vi "Dashboard Main.vi"() -> ()   [LabVIEW 2013]
uses:
  <vilib>/event_ctls.llb/eventvkey.ctl
  <vilib>/Rock Robotics/WPI/Dashboard/WPI_DashboardLogging Global.vi
  <vilib>/Utility/config.llb/Write Key (String).vi
  <vilib>/Utility/config.llb/Write Key (I32).vi
  <vilib>/Utility/config.llb/NI_LVConfig.lvlib
panel:
  out "Image Message":string="Timeout in Camera Communications"
  in  "Rec Mode":enum32{"Stop", "Record", "Playback"}(radio)
  in  "Dashboard Tab":enum32{"Main", "Test", "Checklist", "Variables"}(tab)
  in  "Camera Settings":T1={"Frame Rate"=30, "Compression"=30, "Size"=1} {"Frame Rate" scale=1.0..30.0; "Size" items=["640x480", "320x240", "160x120"]}
  out "Mode":T2(ring)=enum."Auto Disabled"
  out "Camera IP":string
  in  "DB Camera Config":bool
  out "fps":dbl format="%#.1g"
  out "Mbps":dbl format="%#.1g"
  out "Mbps 2":bool
  in  "Test Slider":dbl(slide) scale=0.0..100.0 scale format="%#_3g"
  in  "On/Off":bool caption="Solenoid"
  in  "Test Name":u16(ring) items=["Select the test to run...", "Example Test", "-------------------------------", "List of tests is built in robot code.", "Replace with your own automated tests."]
  in  "Test Tree":string(tree)
  in  "Motor":cluster{"Value":dbl, "Enable":bool} {"Value" scale=-1.0..1.0 scale format="%#_3g"}
  out "Progress":T3 {"Test Progress" scale=0.0..100.0}
  in  "Rev/Fwd":cluster{"Forward":bool, "Reverse":bool}
  in  "Test Ring":u16(ring) items=["Auto", "Fixed indoor", "Fixed outdoor 1", "Fixed outdoor 2", "Fixed fluorescent 1", "Fixed fluorescent 2", "Hold current"]
  in  "Listbox":i32(listbox)
  out "Tree":string(tree)
  out "Camera Image":T4(plugin-control)
  in  "Enable":bool
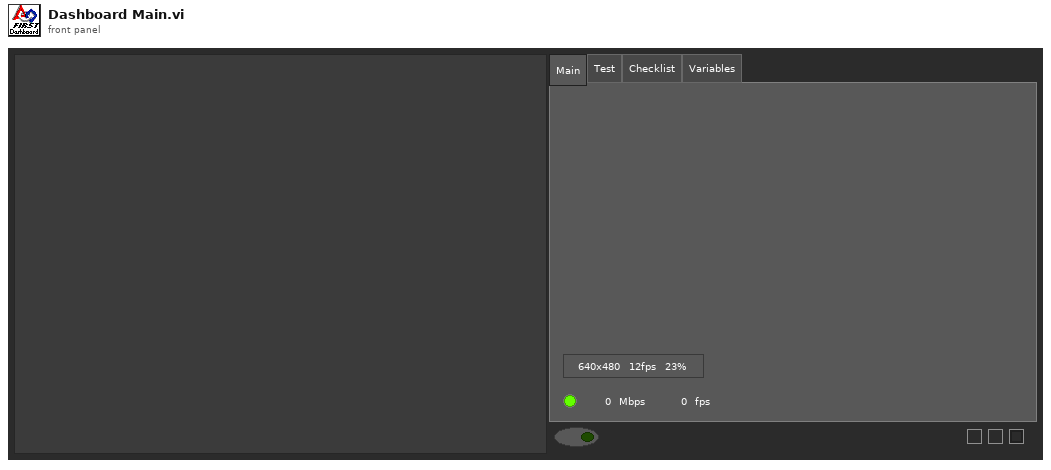
[diagram p1: front panel]
types:
  T1 = cluster{"Frame Rate":i32, "Compression":i32, "Size":u16}
  T2 = enum8{"Tele-Op Disabled", "Tele-Op Enabled", "Auto Disabled", "Auto Enabled", "Test Disabled", "Test Enabled", ""}
  T3 = cluster{"Test Progress":u8, "Test Progress Text":string}
  T4 = typedef "IMAQ Image.ctl" = refnum<image>
  T5 = enum32{"Drive", "Operation", "Auto", "Test", "Checklist", "Variables"}
  T6 = typedef "Image Type" = u32
  T7 = cluster{"Left":i32, "Top":i32, "Right":i32, "Bottom":i32}
  T8 = cluster{"Digital Inputs":bool[], "Digital Outputs":bool[]}
  T9 = cluster{"Competition mode":bool, "Robot Link":bool, "Autonomous":bool, "Enabled":bool, "E-Stop":bool, "Simulated":bool, "TestMode":bool, "Docked Window":bool}
  T10 = typedef "NI_LVConfig.lvlib/Config Data RefNum.ctl" = refnum<k1>
  T11 = typedef "eventvkey.ctl" = enum16{"ASCII", "Enter", "Return", "Shift", "Ctrl", "Alt", "Cmd", "Opt", "Caps", "NumLock", "Clear", "Break", "Up", "Down", "Left", "Right", "Insert", "Delete", "Home", "End", "PageUp", "PageDown", "Escape", "Help", "Pause", "ScrollLock", "F1", "F2", "F3", "F4", "F5", "F6", "F7", "F8", "F9", "F10", "F11", "F12", "F13", "F14", "F15", "F16", "F17", "F18", "F19", "F20", "F21", "F22", "F23", "F24", "Play", "VolumeUp", "VolumeDown", "Mute", "Two Byte Char"}
  T12 = cluster{"Image Size":bool, "Image Type":bool, "Pixel Value":bool, "ROI Information":bool, "Zoom Factor":bool}
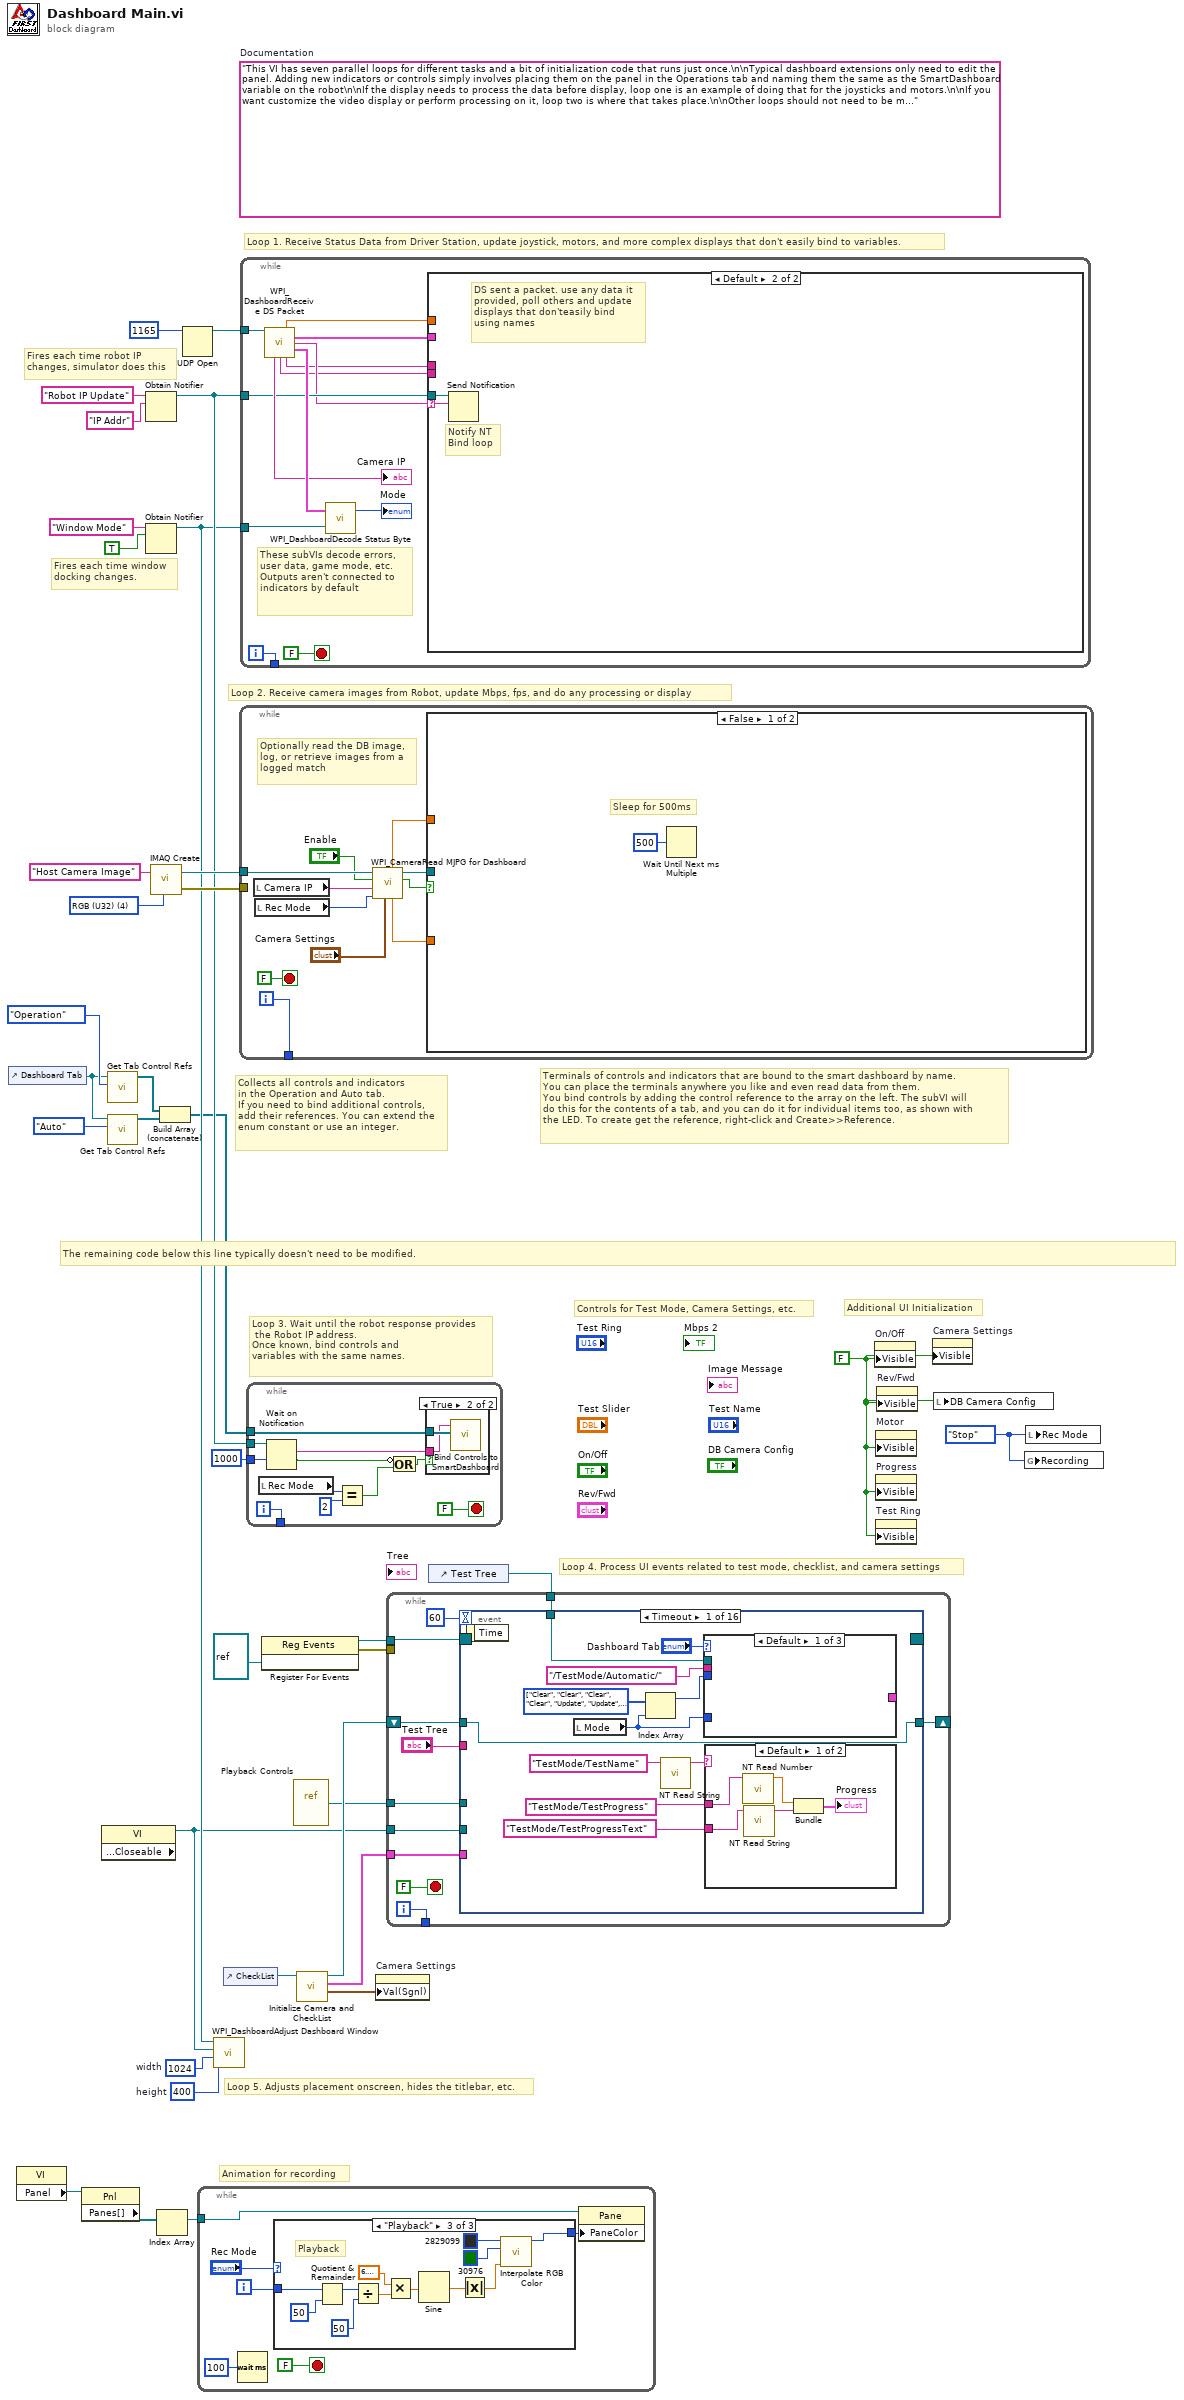
[diagram p0: block diagram]
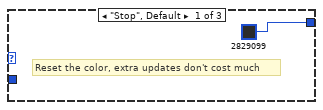
[diagram p2: hidden frame]
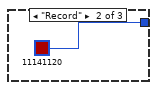
[diagram p3: hidden frame]
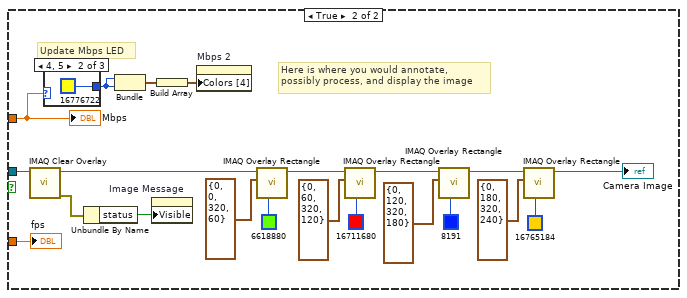
[diagram p5: hidden frame]
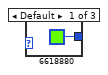
[diagram p6: hidden frame]
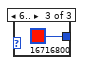
[diagram p7: hidden frame]
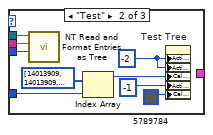
[diagram p8: hidden frame]
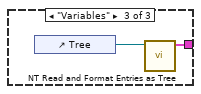
[diagram p9: hidden frame]
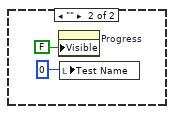
[diagram p10: hidden frame]
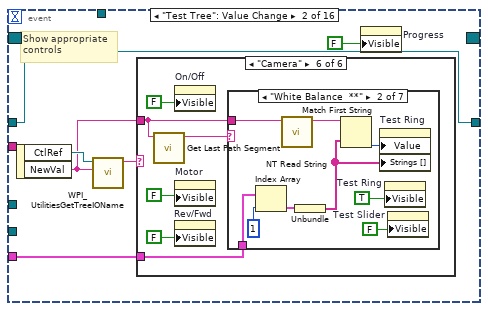
[diagram p11: hidden frame]
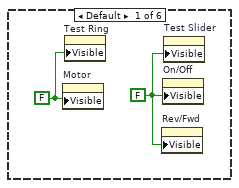
[diagram p12: hidden frame]
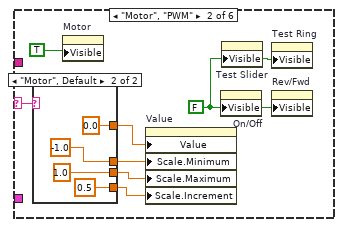
[diagram p13: hidden frame]
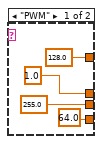
[diagram p14: hidden frame]
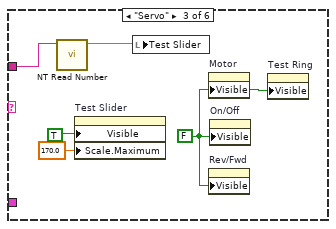
[diagram p15: hidden frame]
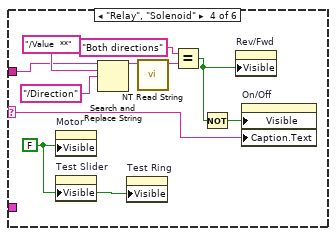
[diagram p16: hidden frame]
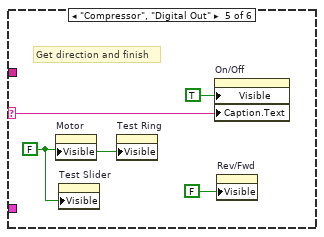
[diagram p17: hidden frame]
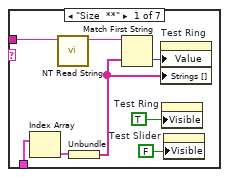
[diagram p18: hidden frame]
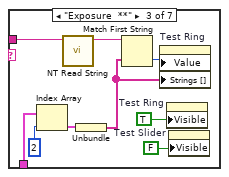
[diagram p19: hidden frame]
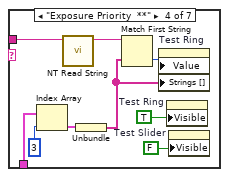
[diagram p20: hidden frame]
diagram:
  w7 = enum32{"Stop", "Record", "Playback"}."Stop" ("Rec Mode")
  w10 = 400  # height
  w11 = 1024  # width
  w24 = FALSE ("Visible")
  (unwired) "This VI has seven parallel loops for different tasks and a bit of initialization code that runs just once.\n\nTypical dashboard extensions only need to edit the panel. Adding new indicators or controls simply involves placing them on the panel in the Operations tab and naming them the same as the SmartDashboard variable on the robot\n\nIf the display needs to process the data before display, loop one is an example of doing that for the joysticks and motors.\n\nIf you want customize the video display or perform processing on it, loop two is where that takes place.\n\nOther loops should not need to be modified. They are pretty standard, and document the task they perform."  # Documentation
  w34 = T6 4 items=["Grayscale (U8)", "Grayscale (I16)", "Grayscale (SGL)", "Complex (CSG)", "RGB (U32)", "HSL (U32)", "RGB (U64)"] ("Image Type")
  # "Controls for Test Mode, Camera Settings, etc."
  # "Additional UI Initialization"
  # "Animation for recording"
  # "Fires each time robot IP\nchanges, simulator does this"
  # "Fires each time window\ndocking changes."
  # "Collects all controls and indicators\nin the Operation and Auto tab.\nIf you need to bind additional controls,\nadd their references. You can extend the\nenum constant or use an integer."
  # "The remaining code below this line typically doesn't need to be modified."
  # "Loop 4. Process UI events related to test mode, checklist, and camera settings"
  # "Terminals of controls and indicators that are bound to the smart dashboard by name.\nYou can place the terminals anywhere you like and even read data from them.\nYou bind controls by adding the control reference to the array on the left. The subVI will\ndo this for the contents of a tab, and you can do it for individual items too, as shown with\nthe LED. To create get the reference, right-click and Create>>Reference."
  # "Loop 3. Wait until the robot response provides\n the Robot IP address.\nOnce known, bind controls and\nvariables with the same names."
  # "Loop 5. Adjusts placement onscreen, hides the titlebar, etc."
  # "Loop 1. Receive Status Data from Driver Station, update joystick, motors, and more complex displays that don't easily bind to variables."
  # "Loop 2. Receive camera images from Robot, update Mbps, fps, and do any processing or display"
  n1 = control-ref of="Dashboard Tab"() -> (w5:refnum<vi>)
  n2 = property class="VI"() -> ("Panel"=w18:refnum<vi>)  [unwired: 2 in, 2 out]
  n3 = property class="Pnl"(reference=w18) -> ("Panes[]"=w19:refnum<vi>[])  [unwired: 1 in, 2 out]
  n4 = property class="VI" props=["Front Panel.Closeable"]() -> (reference out=w6:refnum<vi>)  [unwired: 2 in, 2 out]
  n5 = call <vilib>:"Get Tab Control Refs.vi"("Page Index"=T5."Operation" ("Dashboard Tab"), "TabControl in"=w5) -> ("ControlsOnPage"=w3:refnum<vi>[])  [unwired: 9 in]
  n6 = call <vilib>:"Get Tab Control Refs.vi"("Page Index"=T5."Auto" ("Dashboard Tab"), "TabControl in"=w5) -> ("ControlsOnPage"=w4:refnum<vi>[])  [unwired: 9 in]
  n7 = Obtain Notifier(name (unnamed)="Robot IP Update", notification data type="IP Addr" ("name (unnamed)")) -> (notifier out=w28:refnum<notifier>)  [unwired: 2 in, 2 out]
  n8 = Obtain Notifier(name (unnamed)="Window Mode", notification data type=TRUE) -> (notifier out=w9:refnum<notifier>)  [unwired: 2 in, 2 out]
  n9 = call "IMAQ Create"("Image Name"="Host Camera Image", "Image Type"=w34) -> ("New Image"=w32:T4, "error out"=w31:errorcluster)  [unwired: 2 in, 1 out]
  n10 = Index Array(array=w19) -> (element=w17:refnum<vi>)  [unwired: 1 in]
  n11 = Build Array (concatenate)(w3, w4) -> (w2:refnum<vi>[])
  n12 = UDP Open(11:u16 1165 ("port")) -> (port=w35:refnum<k16>)  [unwired: 2 in, 4 out]
  n13 = while {
    tunnel: w17 -> [w38]
    i -> [w41]
    stop <- FALSE stop-if-true
    n14 = Wait (ms)(milliseconds to wait=u32 100) -> ()  [unwired: 1 out]
    n15 = case shown="\"Playback\"" "Rec Mode" {
      tunnel: w41 -> [_ _ w56]
      tunnel: [u32 2829099 ("Base Color") u32 11141120 ("Target Color") w45] -> w37
      frame "Stop", Default {
        # "Reset the color, extra updates don't cost much"
      }
      frame "Record" {
      }
      frame "Playback" {
        # "Playback"
        n16 = Quotient & Remainder(x=w56, y=u32 50 ("milliseconds to wait")) -> (x-y*floor(x/y)=w52:u32)  [unwired: 1 out]
        n17 = Divide(x=w52, y=u32 50 ("milliseconds to wait")) -> (x/y=w49:dbl)
        n18 = Multiply(x=6.283185307179586, y=w49) -> (x*y=w54:dbl)
        n19 = Sine(x=w54) -> (sin(x)=w53:dbl)
        n20 = Absolute Value(x=w53) -> (abs(x)=w46:dbl)
        n21 = call "Interpolate RGB Color.vi"("Proportion"=w46, "Target Color"=u32 30976, "Base Color"=u32 2829099) -> ("Result Color"=w45:u32)  [unwired: 8 in]
      }
    }
    n22 = property class="Pane"(reference=w38, "PaneColor"=w37) -> ()  [unwired: 1 in, 2 out]
  }
  n23 = call <vilib>:"WPI_DashboardAdjust Dashboard Window.vi"("height"=w10, "width"=w11, "reference in"=w6, "Notifier in"=w9) -> ()  [unwired: 8 in]
  n24 = control-ref of="CheckList"() -> (w8:refnum<vi>)
  n25 = while {
    tunnel: w32 -> [w65]
    tunnel: w31 -> [_]
    tunnel: [w66] -> _
    i -> [w66]
    stop <- FALSE stop-if-true
    # "Optionally read the DB image,\nlog, or retrieve images from a\nlogged match"
    n26 = local read "Camera IP"() -> (w59:string)
    n27 = local read "Rec Mode"() -> (w58:enum32{"Stop", "Record", "Playback"})
    n28 = call <vilib>:"WPI_CameraRead MJPG for Dashboard.vi"("Camera Settings"="Camera Settings", "Rec Mode"=w58, "Camera IP"=w59, "Enable"="Enable", "Refnum in"=w65) -> ("Active"=w57:bool, "Refnum out"=w64:T4, "FPS"=w62:dbl, "Bandwidth (Mbps)"=w61:dbl)  [unwired: 3 in]
    n29 = case shown="False" w57 {
      tunnel: w64 -> [_ w84]
      tunnel: w61 -> [_ w83]
      tunnel: w62 -> [_ w82]
      frame False {
        # "Sleep for 500ms"
        n30 = Wait Until Next ms Multiple(millisecond multiple=u32 500) -> ()  [unwired: 1 out]
      }
      frame True {
        # "Here is where you would annotate,\npossibly process, and display the image"
        # "Update Mbps LED"
        n31 = call "IMAQ Clear Overlay"("Image"=w84) -> ("error out"=w88:errorcluster, "Image Out"=w81:T4)  [unwired: 2 in, 7 out]
        n32 = case shown="4, 5" w83 {
          tunnel: [u32 6618880 ("Color Box") u32 16776722 ("Color Box") u32 16716800 ("Color Box")] -> w85
          frame Default {
          }
          frame 4, 5 {
          }
          frame 6.. {
          }
        }
        n33 = Unbundle By Name(w88) -> ("status"=w89:bool)
        n34 = Bundle("Color Box"=w85, "Color Box"=w85) -> (w87:cluster{"Color Box":u32, "Color Box":u32})  [unwired: 1 out]
        n35 = property on="Image Message" class="Str"("Visible"=w89) -> ()  [unwired: 2 in, 2 out]
        n36 = Build Array(w87) -> (w86:cluster{"Color Box":u32, "Color Box":u32}[])
        n37 = property on="Mbps 2" class="Bool (strict)"("Colors [4]"=w86) -> ()  [unwired: 2 in, 2 out]
        n38 = call "IMAQ Overlay Rectangle"("Color"=u32 6618880, "Rectangle"=T7 {"Left"=0, "Top"=0, "Right"=320, "Bottom"=60}, "Image"=w81) -> ("Image Out"=w80:T4)  [unwired: 7 in, 1 out]
        n39 = call "IMAQ Overlay Rectangle"("Color"=u32 16711680, "Rectangle"=T7 {"Left"=0, "Top"=60, "Right"=320, "Bottom"=120}, "Image"=w80) -> ("Image Out"=w79:T4)  [unwired: 7 in, 1 out]
        n40 = call "IMAQ Overlay Rectangle"("Color"=u32 8191, "Rectangle"=T7 {"Left"=0, "Top"=120, "Right"=320, "Bottom"=180}, "Image"=w79) -> ("Image Out"=w78:T4)  [unwired: 7 in, 1 out]
        n41 = call "IMAQ Overlay Rectangle"("Color"=u32 16765184, "Rectangle"=T7 {"Left"=0, "Top"=180, "Right"=320, "Bottom"=240}, "Image"=w78) -> ("Image Out"=→"Camera Image":T4)  [unwired: 7 in, 1 out]
        "Mbps" <- w83
        "fps" <- w82
      }
    }
  }
  n42 = while {
    tunnel: w35 -> [w103]
    tunnel: w28 -> [w98]
    tunnel: w9 -> [w102]
    tunnel: [w99] -> _
    i -> [w99]
    stop <- FALSE stop-if-true
    # "These subVIs decode errors, user data, game mode, etc.\nOutputs aren't connected to indicators by default"
    n43 = call <vilib>:"WPI_DashboardReceive DS Packet.vi"("Recv Socket"=w103) -> ("Battery"=w93:sgl, "Driver Station"=w94:T8, "Robot IP Address"=w97:string, "Status"=w104:T9, "Camera IP Address"=→"Camera IP":string, "Low Priority User Data"=w96:string, "High Priority User Data"=w95:string)  [unwired: 1 in, 7 out]
    n44 = call <vilib>:"WPI_DashboardDecode Status Byte.vi"("Window Mode Notifier"=w102, "Status"=w104) -> ("Mode"=→"Mode":T2)  [unwired: 1 out]
    n45 = case shown="Default" w97 {
      selector: w97 -> [_ w106]
      tunnel: w98 -> [_ w107]
      tunnel: w96 -> [_ _]
      tunnel: w95 -> [_ _]
      tunnel: w94 -> [_ _]
      tunnel: w93 -> [_ _]
      frame "0.0.0.0" {
        # "DS not sending packets, or no robot exists yet.\nDon't poll the variables"
      }
      frame Default {
        # "Notify NT\nBind loop"
        # "DS sent a packet. use any data it\nprovided, poll others and update\ndisplays that don'teasily bind\nusing names"
        n46 = Send Notification(notification=w106, notifier=w107) -> ()  [unwired: 1 in, 2 out]
      }
    }
  }
  n47 = while {
    tunnel: w2 -> [w118]
    tunnel: w28 -> [w116]
    tunnel: [w114] -> _
    tunnel: u32 1000 ("milliseconds to wait") -> [w113]
    i -> [w114]
    stop <- FALSE stop-if-true
    n48 = local read "Rec Mode"() -> (w109:enum32{"Stop", "Record", "Playback"})
    n49 = Wait on Notification(notifier=w116, timeout in ms (-1)=w113) -> (notification=w115:string, timed out?=w111:bool)  [unwired: 2 in, 2 out]
    n50 = Equal?(x=w109, y=u16 2 ("Rec Mode")) -> (x = y?=w110:bool)
    n51 = Compound Arithmetic op=OR(invert w111, w110) -> (w112:bool)
    n52 = case shown="True" w112 {
      tunnel: w118 -> [_ w120]
      tunnel: w115 -> [_ w119]
      frame False {
      }
      frame True {
        n53 = call <vilib>:"Bind Controls to SmartDashboard.vi"("Bound Control Refs"=w120, "Server IP Address"=w119) -> ()  [unwired: 10 in]
      }
    }
  }
  n54 = register-events(refnum<vi> refnum) -> (reference out=w15:refnum<event-registration>, error out=w14:errorcluster)  [unwired: 2 in]
  n55 = vi-ref "Playback Controls.vi"() -> (w16:refnum<vi>)
  n56 = call "Initialize Camera and CheckList.vi"("ListBox in"=w8) -> ("Cluster"=w22:cluster{"value":i32, "value":i32, "index":i32}, "Array"=w23:cluster{string[]}[], "File Refnum"=w21:T10)  [unwired: 8 in]
  n57 = property on="Camera Settings" class="Clust (strict)"("Val(Sgnl)"=w22) -> ()  [unwired: 2 in, 2 out]
  n58 = control-ref of="Test Tree"() -> (w20:refnum<vi>)
  n59 = while {
    tunnel: w23 -> [w128]
    shift-right: [w127] -> _
    shift-left: w21 -> [w126]
    tunnel: [w125] -> _
    tunnel: w20 -> [w124]
    tunnel: w16 -> [w123]
    tunnel: w15 -> [w122]
    tunnel: w14 -> [_]
    tunnel: w6 -> [w121]
    i -> [w125]
    stop <- FALSE stop-if-true
    n60 = event shown="[0] Timeout" {
      selector: w122 -> [_ _ _ _ _ _ _ _ _ _ _ _ _ _ _ _]
      dyn-events: [_ _ _ _ _ _ _ _ _ _ _ _ _ w366 _ _] -> _
      timeout: u32 60 ("milliseconds to wait") -> [_ _ _ _ _ _ _ _ _ _ _ _ _ _ _ _]
      tunnel: w124 -> [w138 _ _ _ _ _ _ _ _ _ _ _ _ _ _ _]
      tunnel: "Test Tree" -> [_ _ _ _ _ _ _ _ w335 w343 w345 w349 w357 _ _ _]
      tunnel: w128 -> [_ w162 _ _ _ _ w299 w329 _ _ _ _ _ _ _ _]
      tunnel: [w132 w161 w260 w265 w273 w285 w298 w322 w334 w341 w344 w348 w356 w368 w382 w383] -> w127
      tunnel: w126 -> [w132 w161 w260 w265 w273 w285 w297 w322 w334 w341 w344 w348 w356 w368 w382 w383]
      tunnel: w123 -> [_ _ _ _ _ _ _ _ _ _ _ _ _ w369 _ w386]
      tunnel: w121 -> [_ _ _ _ _ _ _ _ _ _ _ _ _ w364 _ _]
      event Timeout {
        w137 = enum16{"Update", "Clear"}[] [enum."Clear", enum."Clear", enum."Clear", enum."Clear", enum."Update", enum."Update", enum."Clear"] items=["Update", "Clear"]
        n61 = event-data() -> ()  [unwired: 1 in, 1 out]
        n62 = local read "Mode"() -> (w135:T2)
        n63 = Index Array(array=w137, index=w135) -> (element=w136:enum16{"Update", "Clear"})
        n64 = call <vilib>:"NT Read String.vi"("Name"="TestMode/TestName") -> ("String"=w141:string)  [unwired: 9 in, 1 out]
        n65 = case shown="Default" "Dashboard Tab" {
          tunnel: w138 -> [_ w151 _]
          tunnel: "/TestMode/Automatic/" ("Name Pattern") -> [_ w150 _]
          tunnel: w136 -> [_ w149 _]
          tunnel: w135 -> [_ w147 _]
          tunnel: [_ _ w153] -> _
          frame Default {
          }
          frame "Test" {
            w146 = -2 ("Active Item:Row Number")
            n66 = call <vilib>:"NT Read and Format Entries as Tree.vi"("Operation"=w149, "Name Pattern"=w150, "Tree Refnum"=w151) -> ()  [unwired: 7 in, 2 out]
            n67 = Index Array(array=u32[] [14013909, 14013909, 14013909, 14013909, 14013909, 16777215, 14013909], index=w147) -> (element=w145:u32)
            n68 = property on="Test Tree" class="Tree (strict)"("Active Item Row Number"=w146, "ActiveColNum"=w146, "CellBG"=w145, "Active Item Row Number"=-1 ("Active Item:Row Number"), "CellBG"=u32 5789784 ("Color Box")) -> ()  [unwired: 2 in, 2 out]
          }
          frame "Variables" {
            n69 = control-ref of="Tree"() -> (w152:refnum<vi>)
            n70 = call <vilib>:"NT Read and Format Entries as Tree.vi"("Tree Refnum"=w152) -> ("Formatted Strings"=w153:cluster{"Name":string, "Value":string}[])  [unwired: 9 in, 1 out]
          }
        }
        n71 = case shown="Default" w141 {
          tunnel: "TestMode/TestProgress" ("Name") -> [w155 _]
          tunnel: "TestMode/TestProgressText" ("Name") -> [w154 _]
          frame Default {
            n72 = call <vilib>:"NT Read Number.vi"("Name"=w155) -> ("Numeric"=w156:dbl)  [unwired: 9 in, 1 out]
            n73 = call <vilib>:"NT Read String.vi"("Name"=w154) -> ("String"=w157:string)  [unwired: 9 in, 1 out]
            n74 = Bundle("Numeric"=w156, "String"=w157) -> (→"Progress":cluster{"Numeric":dbl, "String":string})  [unwired: 1 in]
          }
          frame "" {
            n75 = property on="Progress" class="Clust (strict)"("Visible"=FALSE) -> ()  [unwired: 2 in, 2 out]
            n76 = local write "Test Name"(u16 0) -> ()
          }
        }
      }
      event "Test Tree": Value Change {
        # "Show appropriate\ncontrols"
        n77 = event-data() -> ("CtlRef"=w165:refnum<vi>, "NewVal"=w163:string)  [unwired: 1 in]
        n78 = call <vilib>:"WPI_UtilitiesGetTreeIOName.vi"("NewVal"=w163, "TreeControl in"=w165) -> ("I/O Name"=w166:string)  [unwired: 9 in]
        n79 = case shown="\"Camera\"" w166 {
          selector: w166 -> [_ w173 _ w191 w200 _]
          tunnel: w163 -> [_ _ w188 w190 _ w207]
          tunnel: w162 -> [_ _ _ _ _ w206]
          frame Default {
            w168 = FALSE ("Visible")
            w167 = FALSE ("Visible")
            n80 = property on="Motor" class="Clust (strict)"("Visible"=w167) -> ()  [unwired: 2 in, 2 out]
            n81 = property on="Test Ring" class="Ring (strict)"("Visible"=w167) -> ()  [unwired: 2 in, 2 out]
            n82 = property on="Rev/Fwd" class="Clust (strict)"("Visible"=w168) -> ()  [unwired: 2 in, 2 out]
            n83 = property on="On/Off" class="Bool (strict)"("Visible"=w168) -> ()  [unwired: 2 in, 2 out]
            n84 = property on="Test Slider" class="Slide (strict)"("Visible"=w168) -> ()  [unwired: 2 in, 2 out]
          }
          frame "Motor", "PWM" {
            w174 = FALSE ("Visible")
            n85 = case shown="\"Motor\", Default" w173 {
              tunnel: [1.0 ("Value") -1.0 ("Value")] -> w172
              tunnel: [255.0 ("Value") 1.0 ("Value")] -> w171
              tunnel: [128.0 ("Value") 0.0 ("Value")] -> w170
              tunnel: [64.0 ("Value") 0.5 ("Value")] -> w169
              frame "PWM" {
              }
              frame "Motor", Default {
              }
            }
            n86 = property on="Motor" class="Clust (strict)"("Visible"=TRUE) -> ()  [unwired: 2 in, 2 out]
            n87 = property on="Value" class="Slide (strict)"("Value"=w170, "Scale.Minimum"=w172, "Scale.Maximum"=w171, "Scale.Increment"=w169) -> ()  [unwired: 2 in, 2 out]
            n88 = property on="On/Off" class="Bool (strict)"("Visible"=w174) -> ()  [unwired: 2 in, 2 out]
            n89 = property on="Test Slider" class="Slide (strict)"("Visible"=w174) -> ()  [unwired: 2 in, 2 out]
            n90 = property on="Test Ring" class="Ring (strict)"("Visible"=w174) -> ()  [unwired: 2 in, 2 out]
            n91 = property on="Rev/Fwd" class="Clust (strict)"("Visible"=w174) -> ()  [unwired: 2 in, 2 out]
          }
          frame "Servo" {
            w186 = FALSE ("Visible")
            n92 = call <vilib>:"NT Read Number.vi"("Name"=w188) -> ("Numeric"=w187:dbl)  [unwired: 9 in, 1 out]
            n93 = property on="Test Slider" class="Slide (strict)"("Visible"=TRUE, "Scale.Maximum"=170.0 ("Scale.Range:Maximum")) -> ()  [unwired: 2 in, 2 out]
            n94 = local write "Test Slider"(w187) -> ()
            n95 = property on="Motor" class="Clust (strict)"("Visible"=w186) -> ()  [unwired: 2 in, 2 out]
            n96 = property on="Rev/Fwd" class="Clust (strict)"("Visible"=w186) -> ()  [unwired: 2 in, 2 out]
            n97 = property on="On/Off" class="Bool (strict)"("Visible"=w186) -> ()  [unwired: 2 in, 2 out]
            n98 = property on="Test Ring" class="Ring (strict)"("Visible"=w186) -> ()  [unwired: 2 in, 2 out]
          }
          frame "Relay", "Solenoid" {
            w189 = FALSE ("Visible")
            n99 = property on="Motor" class="Clust (strict)"("Visible"=w189) -> ()  [unwired: 2 in, 2 out]
            n100 = property on="Test Slider" class="Slide (strict)"("Visible"=w189) -> ()  [unwired: 2 in, 2 out]
            n101 = Search and Replace String(input string=w190, search string="/Value  **", replace string="/Direction") -> (result string=w196:string)  [unwired: 5 in, 3 out]
            n102 = property on="Test Ring" class="Ring (strict)"("Visible"=w189) -> ()  [unwired: 2 in, 2 out]
            n103 = call <vilib>:"NT Read String.vi"("Name"=w196) -> ("String"=w194:string)  [unwired: 9 in, 1 out]
            n104 = Equal?(x="Both directions", y=w194) -> (x = y?=w192:bool)
            n105 = Not(x=w192) -> (.not. x?=w193:bool)
            n106 = property on="Rev/Fwd" class="Clust (strict)"("Visible"=w192) -> ()  [unwired: 2 in, 2 out]
            n107 = property on="On/Off" class="Bool (strict)"("Visible"=w193, "Caption.Text"=w191) -> ()  [unwired: 2 in, 2 out]
          }
          frame "Compressor", "Digital Out" {
            w199 = FALSE ("Visible")
            # "Get direction and finish"
            n108 = property on="Motor" class="Clust (strict)"("Visible"=w199) -> ()  [unwired: 2 in, 2 out]
            n109 = property on="Test Slider" class="Slide (strict)"("Visible"=w199) -> ()  [unwired: 2 in, 2 out]
            n110 = property on="Test Ring" class="Ring (strict)"("Visible"=w199) -> ()  [unwired: 2 in, 2 out]
            n111 = property on="On/Off" class="Bool (strict)"("Visible"=TRUE, "Caption.Text"=w200) -> ()  [unwired: 2 in, 2 out]
            n112 = property on="Rev/Fwd" class="Clust (strict)"("Visible"=FALSE) -> ()  [unwired: 2 in, 2 out]
          }
          frame "Camera" {
            n113 = call <vilib>:"Get Last Path Segment.vi"("String in"=w207) -> ("String out"=w208:string)  [unwired: 10 in]
            n114 = property on="On/Off" class="Bool (strict)"("Visible"=FALSE) -> ()  [unwired: 2 in, 2 out]
            n115 = property on="Motor" class="Clust (strict)"("Visible"=FALSE) -> ()  [unwired: 2 in, 2 out]
            n116 = property on="Rev/Fwd" class="Clust (strict)"("Visible"=FALSE) -> ()  [unwired: 2 in, 2 out]
            n117 = case shown="\"White Balance  **\"" w208 {
              tunnel: w207 -> [w214 w223 w232 w241 w250 _ w256]
              tunnel: w206 -> [w212 w220 w229 w238 w247 _ _]
              frame "Size  **" {
                n118 = Index Array(array=w212) -> (element=w211:cluster{string[]})  [unwired: 1 in]
                n119 = call <vilib>:"NT Read String.vi"("Name"=w214) -> ("String"=w213:string)  [unwired: 9 in, 1 out]
                n120 = Unbundle(w211) -> (w209:string[])
                n121 = Match First String(2:w209, 3:w213) -> (0:w210:i32)  [unwired: 1 out]
                n122 = property on="Test Ring" class="Ring (strict)"("Value"=w210, "Strings []"=w209) -> ()  [unwired: 2 in, 2 out]
                n123 = property on="Test Ring" class="Ring (strict)"("Visible"=TRUE) -> ()  [unwired: 2 in, 2 out]
                n124 = property on="Test Slider" class="Slide (strict)"("Visible"=FALSE) -> ()  [unwired: 2 in, 2 out]
              }
              frame "White Balance  **" {
                n125 = Index Array(array=w220, index=1) -> (element=w221:cluster{string[]})
                n126 = call <vilib>:"NT Read String.vi"("Name"=w223) -> ("String"=w222:string)  [unwired: 9 in, 1 out]
                n127 = Unbundle(w221) -> (w218:string[])
                n128 = Match First String(2:w218, 3:w222) -> (0:w217:i32)  [unwired: 1 out]
                n129 = property on="Test Ring" class="Ring (strict)"("Value"=w217, "Strings []"=w218) -> ()  [unwired: 2 in, 2 out]
                n130 = property on="Test Ring" class="Ring (strict)"("Visible"=TRUE) -> ()  [unwired: 2 in, 2 out]
                n131 = property on="Test Slider" class="Slide (strict)"("Visible"=FALSE) -> ()  [unwired: 2 in, 2 out]
              }
              frame "Exposure  **" {
                n132 = Index Array(array=w229, index=2) -> (element=w230:cluster{string[]})
                n133 = call <vilib>:"NT Read String.vi"("Name"=w232) -> ("String"=w231:string)  [unwired: 9 in, 1 out]
                n134 = Unbundle(w230) -> (w226:string[])
                n135 = Match First String(2:w226, 3:w231) -> (0:w227:i32)  [unwired: 1 out]
                n136 = property on="Test Ring" class="Ring (strict)"("Value"=w227, "Strings []"=w226) -> ()  [unwired: 2 in, 2 out]
                n137 = property on="Test Ring" class="Ring (strict)"("Visible"=TRUE) -> ()  [unwired: 2 in, 2 out]
                n138 = property on="Test Slider" class="Slide (strict)"("Visible"=FALSE) -> ()  [unwired: 2 in, 2 out]
              }
              frame "Exposure Priority  **" {
                n139 = Index Array(array=w238, index=3) -> (element=w239:cluster{string[]})
                n140 = call <vilib>:"NT Read String.vi"("Name"=w241) -> ("String"=w240:string)  [unwired: 9 in, 1 out]
                n141 = Unbundle(w239) -> (w235:string[])
                n142 = Match First String(2:w235, 3:w240) -> (0:w236:i32)  [unwired: 1 out]
                n143 = property on="Test Ring" class="Ring (strict)"("Value"=w236, "Strings []"=w235) -> ()  [unwired: 2 in, 2 out]
                n144 = property on="Test Ring" class="Ring (strict)"("Visible"=TRUE) -> ()  [unwired: 2 in, 2 out]
                n145 = property on="Test Slider" class="Slide (strict)"("Visible"=FALSE) -> ()  [unwired: 2 in, 2 out]
              }
              frame "Color Enable  **" {
                n146 = Index Array(array=w247, index=4) -> (element=w248:cluster{string[]})
                n147 = call <vilib>:"NT Read String.vi"("Name"=w250) -> ("String"=w249:string)  [unwired: 9 in, 1 out]
                n148 = Unbundle(w248) -> (w244:string[])
                n149 = Match First String(2:w244, 3:w249) -> (0:w245:i32)  [unwired: 1 out]
                n150 = property on="Test Ring" class="Ring (strict)"("Value"=w245, "Strings []"=w244) -> ()  [unwired: 2 in, 2 out]
                n151 = property on="Test Ring" class="Ring (strict)"("Visible"=TRUE) -> ()  [unwired: 2 in, 2 out]
                n152 = property on="Test Slider" class="Slide (strict)"("Visible"=FALSE) -> ()  [unwired: 2 in, 2 out]
              }
              frame Default {
                n153 = property on="Test Ring" class="Ring (strict)"("Visible"=FALSE) -> ()  [unwired: 2 in, 2 out]
                n154 = property on="Test Slider" class="Slide (strict)"("Visible"=FALSE) -> ()  [unwired: 2 in, 2 out]
              }
              frame "Brightness  **", "Color Level  **", "Compression  **", "FPS  **", "Sharpness  **" {
                n155 = call <vilib>:"NT Read Number.vi"("Name"=w256) -> ("Numeric"=w255:dbl)  [unwired: 9 in, 1 out]
                n156 = local write "Test Slider"(w255) -> ()
                n157 = property on="Test Slider" class="Slide (strict)"("Visible"=TRUE, "Scale.Maximum"=100.0 ("Scale.Range:Maximum")) -> ()  [unwired: 2 in, 2 out]
                n158 = property on="Test Ring" class="Ring (strict)"("Visible"=FALSE) -> ()  [unwired: 2 in, 2 out]
              }
            }
          }
        }
        n159 = property on="Progress" class="Clust (strict)"("Visible"=FALSE) -> ()  [unwired: 2 in, 2 out]
      }
      event "Test Name": Mouse Enter {
        # "Populate the ring with the list of tests"
        n160 = event-data() -> ()  [unwired: 1 in, 1 out]
        n161 = call <vilib>:"NT Read String Array.vi"("Name"="TestMode/TestList") -> ("String Array"=w264:string[])  [unwired: 9 in, 1 out]
        n162 = Build Array (concatenate)("Select the test to run...", w264) -> (w263:string[])
        n163 = property on="Test Name" class="Ring (strict)"("Strings []"=w263) -> ()  [unwired: 2 in, 2 out]
      }
      event "Test Name": Value Change {
        w266 = FALSE ("Visible")
        # "Tell the robot the test name to run"
        n164 = event-data() -> ("NewVal"=w270:u16)  [unwired: 1 in]
        n165 = property on="Test Name" class="Ring (strict)"() -> ("Strings []"=w271:string[])  [unwired: 2 in, 2 out]
        n166 = local write "Progress"(T3 {"Test Progress"=0, "Test Progress Text"=""} ("Progress")) -> ()
        n167 = Index Array(array=w271, index=w270) -> (element=w269:string)
        n168 = call <vilib>:"NT Write String.vi"("String"=w269, "Name"="TestMode/TestName") -> ()  [unwired: 9 in, 1 out]
        n169 = property on="Progress" class="Clust (strict)"("Visible"=TRUE) -> ()  [unwired: 2 in, 2 out]
        n170 = property on="Motor" class="Clust (strict)"("Visible"=w266) -> ()  [unwired: 2 in, 2 out]
        n171 = property on="Test Slider" class="Slide (strict)"("Visible"=w266) -> ()  [unwired: 2 in, 2 out]
        n172 = property on="On/Off" class="Bool (strict)"("Visible"=w266) -> ()  [unwired: 2 in, 2 out]
        n173 = property on="Rev/Fwd" class="Clust (strict)"("Visible"=w266) -> ()  [unwired: 2 in, 2 out]
        n174 = property on="Test Ring" class="Ring (strict)"("Visible"=w266) -> ()  [unwired: 2 in, 2 out]
      }
      event "Listbox": Double Click {
        n175 = event-data() -> ("PlatMods.Shift"=w274:bool, "Row"=w276:i32)  [unwired: 1 in]
        n176 = case shown="True" w274 {
          tunnel: w276 -> [w280 _]
          tunnel: 1 -> [w279 _]
          frame False {
            n177 = property on="Listbox" class="LstBox (strict)"() -> ("Item Symbols"=w278:i32[])  [unwired: 2 in, 2 out]
            n178 = Replace Array Subset(array=w278, new element=w279, index=w280) -> (w277:i32[])
            n179 = property on="Listbox" class="LstBox (strict)"("Item Symbols"=w277) -> ()  [unwired: 2 in, 2 out]
          }
          frame True {
            w281 = 0 ("Top Row")
            n180 = property on="Listbox" class="LstBox (strict)"() -> ("Number of Rows"=w283:u32)  [unwired: 2 in, 2 out]
            n181 = Initialize Array(0, w283) -> (w282:i32[])
            n182 = property on="Listbox" class="LstBox (strict)"("Top Row"=w281, "Value"=w281, "Item Symbols"=w282) -> ()  [unwired: 2 in, 2 out]
          }
        }
      }
      event "Listbox": Key Down {
        n183 = event-data() -> ("VKey"=w287:T11)  [unwired: 1 in]
        n184 = case shown="\"Left\", \"Right\"" w287 {
          selector: w287 -> [w292 _]
          tunnel: eventvkey."Left" ("VKey") -> [w290 _]
          frame "Left", "Right" {
            n185 = Equal?(x=w290, y=w292) -> (x = y?=w291:bool)
            n186 = Select(t=0, s=w291, f=1) -> (s? t:f=w293:i32)
            n187 = property on="Listbox" class="LstBox (strict)"() -> ("Item Symbols"=w296:i32[])  [unwired: 2 in, 2 out]
            n188 = Replace Array Subset(array=w296, new element=w293, index="Listbox") -> (w295:i32[])
            n189 = property on="Listbox" class="LstBox (strict)"("Item Symbols"=w295) -> ()  [unwired: 2 in, 2 out]
          }
          frame Default {
          }
        }
      }
      event "DB Camera Config": Value Change {
        n190 = event-data() -> ("NewVal"=w300:bool)  [unwired: 1 in]
        n191 = case shown="False" w300 {
          tunnel: w299 -> [w309 _]
          tunnel: [w302 w320] -> w298
          tunnel: w297 -> [w301 w320]
          frame False {
            w316 = "Camera"
            w319 = FALSE ("Visible")
            n192 = local read "Camera Settings"() -> (w308:T1)
            n193 = Index Array(array=w309) -> (element=w312:cluster{string[]})  [unwired: 1 in]
            n194 = Unbundle(w308) -> ("Frame Rate"=w307:i32, "Compression"=w306:i32, "Size"=w310:u16)
            n195 = Unbundle(w312) -> (w311:string[])
            n196 = Index Array(array=w311, index=w310) -> (element=w305:string)
            n197 = call-poly <vilib>:"Write Key.vi"("section"=w316, "value"=w305, "key"="Size", "refnum"=w301) -> ("refnum out"=w318:T10)  [unwired: 2 in, 5 out]
            n198 = call-poly <vilib>:"Write Key.vi"("section"=w316, "value"=w307, "key"="FrameRate", "refnum"=w318) -> ("refnum out"=w317:T10)  [unwired: 1 in, 6 out]
            n199 = property on="Camera Settings" class="Clust (strict)"("Visible"=w319) -> ()  [unwired: 2 in, 2 out]
            n200 = local write "DB Camera Config"(w319) -> ()
            n201 = call-poly <vilib>:"Write Key.vi"("section"=w316, "value"=w306, "key"="Compression", "refnum"=w317) -> ("refnum out"=w303:T10)  [unwired: 1 in, 6 out]
            n202 = call <vilib>:"Close Config Data.vi"("refnum"=w303) -> ("file path"=w304:path)  [unwired: 2 in, 8 out]
            n203 = call <vilib>:"Open Config Data.vi"("configuration file path"=w304) -> ("refnum"=w302:T10)  [unwired: 8 in, 2 out]
          }
          frame True {
            n204 = property on="Camera Settings" class="Clust (strict)"("Visible"=TRUE) -> ()  [unwired: 2 in, 2 out]
          }
        }
      }
      event "Camera Settings": Value Change {
        n205 = event-data() -> ("NewVal"=w333:T1)  [unwired: 1 in]
        n206 = Index Array(array=w329) -> (element=w328:cluster{string[]})  [unwired: 1 in]
        n207 = Unbundle(w333) -> ("Frame Rate"=w324:i32, "Compression"=w323:i32, "Size"=w326:u16)
        n208 = Unbundle(w328) -> (w327:string[])
        n209 = Index Array(array=w327, index=w326) -> (element=w325:string)
        n210 = Format Into String(format string="%s   %dfps   %d%%", w325, w324, w323) -> (resulting string=w330:string)  [unwired: 2 in, 1 out]
        n211 = Build Array(w330) -> (w331:string[])
        n212 = property on="DB Camera Config" class="Bool (strict)"("Strings [4]"=w331) -> ()  [unwired: 2 in, 2 out]
      }
      event "Motor.Enable": Value Change {
        n213 = event-data() -> ("NewVal"=w339:bool)  [unwired: 1 in]
        n214 = Unbundle("Motor") -> ("Value"=w338:dbl)  [unwired: 1 out]
        n215 = Select(t=w338, s=w339, f=0.0) -> (s? t:f=w336:dbl)
        n216 = call <vilib>:"NT Write Number.vi"("Numeric"=w336, "Name"=w335) -> ()  [unwired: 9 in, 1 out]
      }
      event "Test Slider": Value Change {
        n217 = event-data() -> ("NewVal"=w342:dbl)  [unwired: 1 in]
        n218 = call <vilib>:"NT Write Number.vi"("Numeric"=w342, "Name"=w343) -> ()  [unwired: 9 in, 1 out]
      }
      event "On/Off": Value Change {
        n219 = event-data() -> ("NewVal"=w347:bool)  [unwired: 1 in]
        n220 = Boolean To (0,1)(Boolean=w347) -> (0, 1=w346:i16)
        n221 = call <vilib>:"NT Write Number.vi"("Numeric"=w346, "Name"=w345) -> ()  [unwired: 9 in, 1 out]
      }
      event "Rev/Fwd": Value Change {
        n222 = event-data() -> ("NewVal.Forward"=w355:bool, "NewVal.Reverse"=w354:bool)  [unwired: 1 in]
        n223 = Boolean To (0,1)(Boolean=w355) -> (0, 1=w351:i16)
        n224 = Boolean To (0,1)(Boolean=w354) -> (0, 1=w353:i16)
        n225 = Negate(x=w353) -> (-x=w352:i16)
        n226 = Add(x=w351, y=w352) -> (x+y=w350:i16)
        n227 = call <vilib>:"NT Write Number.vi"("Numeric"=w350, "Name"=w349) -> ()  [unwired: 9 in, 1 out]
      }
      event "Test Ring": Value Change {
        n228 = event-data() -> ("NewVal"=w359:u16)  [unwired: 1 in]
        n229 = property on="Test Ring" class="Ring (strict)"() -> ("Strings []"=w360:string[])  [unwired: 2 in, 2 out]
        n230 = Index Array(array=w360, index=w359) -> (element=w358:string)
        n231 = call <vilib>:"NT Write String.vi"("String"=w358, "Name"=w357) -> ()  [unwired: 9 in, 1 out]
      }
      event "Rec Mode": Value Change {
        # "Update globals for recording mode and path to read log from.\nClear when logging and let NetworkTables set path for vision to\nuse."
        n232 = event-data() -> ("NewVal"=w370:enum32{"Stop", "Record", "Playback"})  [unwired: 1 in]
        n233 = global write "WPI_DashboardLogging Global.vi" "Logging Filename"(path "") -> ()
        n234 = case shown="\"Stop\", \"Record\"" w370 {
          tunnel: w369 -> [_ w372 w380]
          tunnel: [_ _ w379] -> w366
          tunnel: [_ _ w378] -> _
          tunnel: w364 -> [_ _ w376]
          tunnel: cluster{i32, i32} {-250, 170} -> [_ _ w375]
          tunnel: [_ _ T12 {"Image Size"=TRUE, "Image Type"=TRUE, "Pixel Value"=TRUE, "ROI Information"=TRUE, "Zoom Factor"=FALSE} ("Image Information Shown:All Elements")] -> w362
          tunnel: [_ _ TRUE ("Zoom Factor")] -> w361
          frame Default {
          }
          frame "Stop", "Record" {
            # "Place Window too"
            n235 = invoke class="VI" method="FP.Close"(reference=w372) -> (reference out=w371:refnum<vi>)  [unwired: 2 in, 2 out]
            n236 = invoke class="VI" method="Abort VI"(reference=w371) -> ()  [unwired: 2 in, 3 out]
          }
          frame "Playback" {
            n237 = call "Open Playback Panel.vi"("Offset"=w375, "DB VI Ref"=w376, "Playback in"=w380) -> ("Playback out"=w377:refnum<vi>)  [unwired: 8 in]
            n238 = register-events(w377) -> (reference out=w379:refnum<event-registration>, error out=w378:errorcluster)  [unwired: 2 in]
          }
        }
        n239 = global write "WPI_DashboardLogging Global.vi" "Recording"(w370) -> ()
        n240 = property on="Camera Image" class="ImageControl"("Image Information Shown"=w362, "Image Information Visible"=w361) -> ()  [unwired: 2 in, 2 out]
        n241 = call <vilib>:"WPI_DashboardNT Log FieldName Cache.vi"("Operation"=enum16{"Lookup/Add", "Index", "Clear"}."Clear") -> ()  [unwired: 8 in, 3 out]
      }
      event Panel Close {
        w381 = enum32{"Stop", "Record", "Playback"}."Stop" ("Rec Mode")
        n242 = event-data() -> ()  [unwired: 1 in, 4 out]
        n243 = local write "Rec Mode"(w381) -> ()
        n244 = global write "WPI_DashboardLogging Global.vi" "Recording"(w381) -> ()
      }
      event Panel Close {
        # "Abort playback window and ourself"
        n245 = event-data() -> ()  [unwired: 1 in, 4 out]
        n246 = invoke class="VI" method="FP.Close"(reference=w386) -> (reference out=w385:refnum<vi>)  [unwired: 2 in, 2 out]
        n247 = invoke class="VI" method="Abort VI"(reference=w385) -> (error out=w384:errorcluster)  [unwired: 2 in, 2 out]
        n248 = invoke class="VI" method="Abort VI"(error in=w384) -> ()  [unwired: 2 in, 3 out]
      }
    }
  }
  n249 = property on="On/Off" class="Bool (strict)"("Visible"=w24) -> ()  [unwired: 2 in, 2 out]
  n250 = property on="Motor" class="Clust (strict)"("Visible"=w24) -> ()  [unwired: 2 in, 2 out]
  n251 = property on="Progress" class="Clust (strict)"("Visible"=w24) -> ()  [unwired: 2 in, 2 out]
  n252 = property on="Test Ring" class="Ring (strict)"("Visible"=w24) -> ()  [unwired: 2 in, 2 out]
  n253 = property on="Rev/Fwd" class="Clust (strict)"("Visible"=w24) -> ()  [unwired: 2 in, 2 out]
  n254 = property on="Camera Settings" class="Clust (strict)"("Visible"=w24) -> ()  [unwired: 2 in, 2 out]
  n255 = local write "DB Camera Config"(w24) -> ()
  n256 = global write "WPI_DashboardLogging Global.vi" "Recording"(w7) -> ()
  n257 = local write "Rec Mode"(w7) -> ()
